vi "set ca mem.vi"(8 "error in":errorcluster, 10 "ca file":string, 11 "lvlibretls configurable context in":refnum<class "lvlibretls configurable context.lvclass">) -> (0 "error out":errorcluster, 3 "lvlibretls configurable context out":refnum<class "lvlibretls configurable context.lvclass">)   [LabVIEW 2016, in "lvlibretls configurable context.lvclass"]
uses:
  lvlibretls configurable context.lvclass
  lvlibretls configurable context.lvclass/lvlibretls configurable context.ctl
  lv tls dll.lvlib
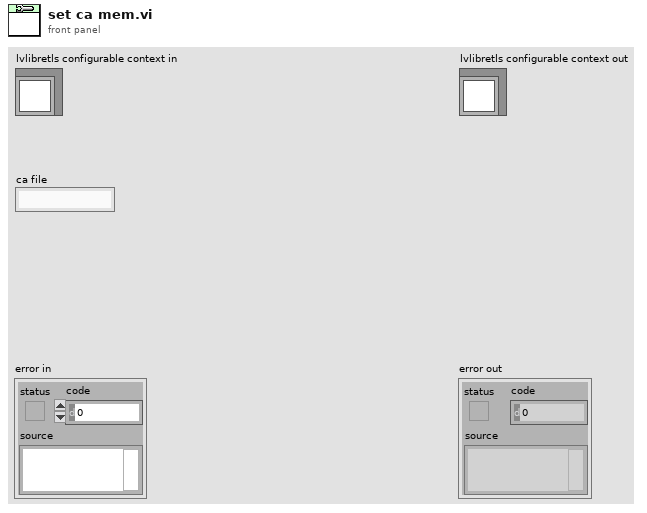
[diagram p1: front panel]
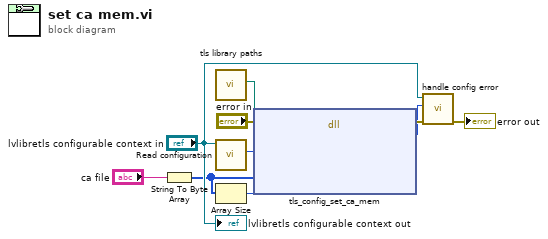
[diagram p0: block diagram]
diagram:
  n1 = String To Byte Array(string="ca file") -> (unsigned byte array=w2:u8[])
  n2 = call "tls library paths.vi"() -> ("libtls"=w10:path)  [unwired: 8 in, 3 out]
  n3 = call "Read configuration.vi"("lvlibretls configurable context in"="lvlibretls configurable context in") -> ("configuration"=w9:u64)  [unwired: 10 in]
  n4 = Array Size(array=w2) -> (size(s)=w1:i32)
  n5 = dll-call lib="C:/Users/IEUser/Desktop/tlssimple/libtls-15.dll" fn="tls_config_set_ca_mem"(path in=w10, error in="error in", "config"=w9, "ca"=w2, "len"=w1) -> (error out=w8:errorcluster, "return"=w7:i32)  [unwired: 4 in, 1 out]
  n6 = call "handle config error.vi"("error in"=w8, "return"=w7, "lvlibretls configurable context in"="lvlibretls configurable context in") -> ("error out"=→"error out":errorcluster)  [unwired: 8 in]
  "lvlibretls configurable context out" <- "lvlibretls configurable context in"
